vi "Interpolate 2D Scattered_Area.vi"(0 "X(Tri) In":dbl[][](array[numeric]), 5 "Y(Tri) In":dbl[][](array[numeric]), 7 "Z(Tri)  In":dbl[][](array[numeric])) -> (4 "X(Tri) Out":dbl[][](array[numeric]), 6 "Y(Tri) Out":dbl[][](array[numeric]), 8 "Z(Tri) Out":dbl[][](array[numeric]), 10 "Area":dbl[](array[numeric]), 15 "Length":dbl[][](array[numeric]))   [LabVIEW 2020, in "NI_AAL_Interpolation.lvlib"]
uses:
  <vilib>/gmath/NI_AAL_Interpolation.lvlib
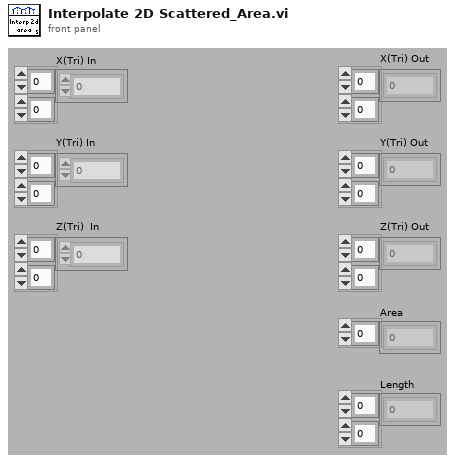
[diagram p1: front panel]
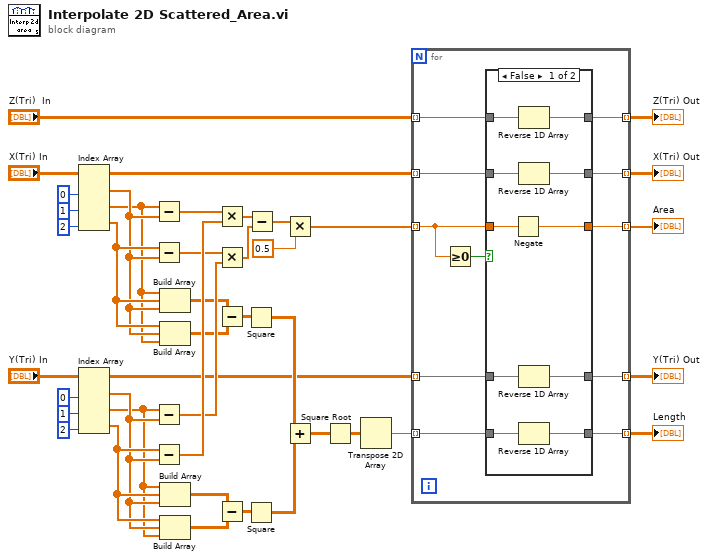
[diagram p0: block diagram]
diagram:
  n1 = Index Array(array="X(Tri) In", index (col) #1=0 ("disabled index (col)"), index (col) #2=1 ("index (col)"), index (col) #3=2 ("index (col)")) -> (element #1=w25:dbl[], element #2=w24:dbl[], element #3=w26:dbl[])  [unwired: 3 in]
  n2 = Index Array(array="Y(Tri) In", index (col) #1=0 ("disabled index (col)"), index (col) #2=1 ("index (col)"), index (col) #3=2 ("index (col)")) -> (element #1=w22:dbl[], element #2=w21:dbl[], element #3=w23:dbl[])  [unwired: 3 in]
  n3 = Subtract(x=w24, y=w25) -> (x-y=w34:dbl[])
  n4 = Subtract(x=w26, y=w25) -> (x-y=w32:dbl[])
  n5 = Subtract(x=w21, y=w22) -> (x-y=w31:dbl[])
  n6 = Subtract(x=w23, y=w22) -> (x-y=w33:dbl[])
  n7 = Build Array(w24, w26, w25) -> (w20:dbl[][])
  n8 = Build Array(w26, w25, w24) -> (w19:dbl[][])
  n9 = Build Array(w21, w23, w22) -> (w18:dbl[][])
  n10 = Build Array(w23, w22, w21) -> (w17:dbl[][])
  n11 = Multiply(x=w34, y=w33) -> (x*y=w30:dbl[])
  n12 = Multiply(x=w32, y=w31) -> (x*y=w29:dbl[])
  n13 = Subtract(x=w20, y=w19) -> (x-y=w16:dbl[][])
  n14 = Subtract(x=w18, y=w17) -> (x-y=w15:dbl[][])
  n15 = Square(x=w16) -> (x^2=w14:dbl[][])
  n16 = Square(x=w15) -> (x^2=w13:dbl[][])
  n17 = Subtract(x=w30, y=w29) -> (x-y=w28:dbl[])
  n18 = Multiply(x=w28, y=0.5) -> (x*y=w10:dbl[])
  n19 = Add(x=w14, y=w13) -> (x+y=w12:dbl[][])
  n20 = Square Root(x=w12) -> (sqrt(x)=w11:dbl[][])
  n21 = Transpose 2D Array(2D array=w11) -> (transposed array=w9:dbl[][])
  n22 = for {
    tunnel: w10 -> [w50] mode=indexing
    tunnel: w9 -> [w42] mode=indexing
    tunnel: "Z(Tri)  In" -> [w47] mode=indexing
    tunnel: "X(Tri) In" -> [w48] mode=indexing
    tunnel: "Y(Tri) In" -> [w49] mode=indexing
    tunnel: [w46] -> w5 mode=indexing
    tunnel: [w45] -> w4 mode=indexing
    tunnel: [w44] -> w3 mode=indexing
    tunnel: [w43] -> w2 mode=indexing
    tunnel: [w41] -> w1 mode=indexing
    n23 = Greater Or Equal To 0?(x=w50) -> (x >= 0?=w51:bool)
    n24 = case shown="False" w51 {
      tunnel: w50 -> [w53 w64]
      tunnel: w49 -> [w55 w63]
      tunnel: w48 -> [w59 w65]
      tunnel: w47 -> [w61 w66]
      tunnel: [w60 w66] -> w46
      tunnel: [w58 w65] -> w45
      tunnel: [w52 w64] -> w44
      tunnel: [w54 w63] -> w43
      tunnel: w42 -> [w57 w62]
      tunnel: [w56 w62] -> w41
      frame False {
        n25 = Negate(x=w53) -> (-x=w52:dbl)
        n26 = Reverse 1D Array(array=w61) -> (reversed array=w60:dbl[])
        n27 = Reverse 1D Array(array=w59) -> (reversed array=w58:dbl[])
        n28 = Reverse 1D Array(array=w55) -> (reversed array=w54:dbl[])
        n29 = Reverse 1D Array(array=w57) -> (reversed array=w56:dbl[])
      }
      frame True {
      }
    }
  }
  "X(Tri) Out" <- w4
  "Y(Tri) Out" <- w2
  "Z(Tri) Out" <- w5
  "Area" <- w3
  "Length" <- w1
